vi "Initialize.vi"(8 "error in":errorcluster, 10 "InstanceName":string, 11 "Chiller Cluster - 1 Channel.lvclass":refnum<class "Device Cluster - 1 Channel.lvclass">) -> (0 "error out":errorcluster, 3 "output cluster":refnum<class "Device Cluster - 1 Channel.lvclass">)   [LabVIEW 2023, in "Device Cluster - 1 Channel.lvclass"]
uses:
  Device Cluster - 1 Channel.lvclass
  Device Cluster - 1 Channel.lvclass/Device Cluster - 1 Channel.ctl
  546b7d5c-4f51-47af-9af1-567894f85656.vi
  397b3e0b-0f1b-47d9-9f6d-8a44e581e150.vi
  546b7d5c-4f51-47af-9af1-567894f85656.vi/4bc1c15b-36ab-481f-b8dd-c64075ce723a.vi
  397b3e0b-0f1b-47d9-9f6d-8a44e581e150.vi/4bc1c15b-36ab-481f-b8dd-c64075ce723a.vi
  <vilib>/ADAS Replay HIL/Channels/Tag Wrapper/Polymorphic/Open Consumer Tag (Cluster).vi
  <vilib>/ADAS Replay HIL/AdasHilServices/AdasHilServices Fill In Error Info Ex.vi
  <vilib>/ADAS Replay HIL/Channels/Tag Wrapper/Polymorphic/Open Producer Tag (Cluster).vi
  Utilities/Utilities.lvlib
  <vilib>/ADAS Replay HIL/Channels/Tag Wrapper/Tag Wrapper.lvlib
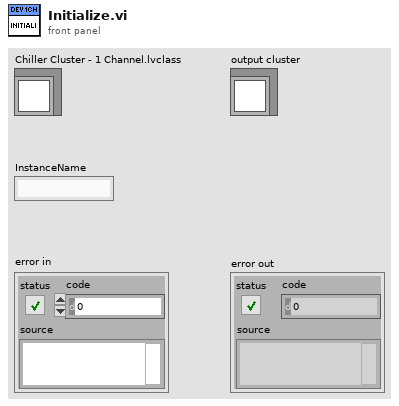
[diagram p1: front panel]
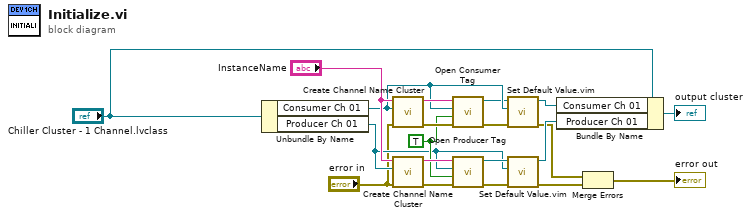
[diagram p0: block diagram]
diagram:
  w10 = TRUE ("Create if not found? (T)")
  n1 = Unbundle By Name("Chiller Cluster - 1 Channel.lvclass") -> ("Consumer Ch 01"=w14:refnum<k21>, "Producer Ch 01"=w9:refnum<k21>)
  n2 = call "Create Channel Name Cluster.vi"("error in"="error in", "Cluster"=w14, "Instance Name"="InstanceName") -> ("error out"=w11:errorcluster, "Data Channel Name"=w17:string)  [unwired: 7 in]
  n3 = call "Create Channel Name Cluster.vi"("error in"="error in", "Cluster"=w9, "Instance Name"="InstanceName") -> ("error out"=w7:errorcluster, "Data Channel Name"=w16:string)  [unwired: 7 in]
  n4 = call-poly <vilib>:"Open Consumer Tag.vi"("error in"=w11, "Create if not found? (T)"=w10, "Cluster"=w14, "Channel Name"=w17) -> ("error out"=w12:errorcluster, "ADAS HIL Channel"=w13:refnum<k21>)  [unwired: 6 in]
  n5 = call-poly <vilib>:"Open Producer Tag.vi"("error in"=w7, "Create if not found? (T)"=w10, "Cluster"=w9, "Channel Name"=w16) -> ("error out"=w8:errorcluster, "ADAS HIL Channel"=w15:refnum<k21>)  [unwired: 6 in]
  n6 = call "Set Default Value.vim"("error in"=w12, "Data in"=w14, "ADAS HIL Channel in"=w13) -> ("error out"=w3:errorcluster, "ADAS HIL Channel out"=w6:refnum<k21>)  [unwired: 7 in]
  n7 = call "Set Default Value.vim"("error in"=w8, "Data in"=w9, "ADAS HIL Channel in"=w15) -> ("error out"=w2:errorcluster, "ADAS HIL Channel out"=w5:refnum<k21>)  [unwired: 7 in]
  n8 = Bundle By Name(cluster="Chiller Cluster - 1 Channel.lvclass", "Consumer Ch 01"=w6, "Producer Ch 01"=w5) -> (→"output cluster":refnum<class "Device Cluster - 1 Channel.lvclass">)
  n9 = Merge Errors(w3, w2) -> (→"error out":errorcluster)
